vi "MP-285 GetSet Resolution.vi"(0 "VISA resource name":refnum<visa-resource-name>, 1 "Input: Resolution - H/L":string="\r", 2 "error in (no error)":errorcluster) -> (3 "VISA resource name 2":refnum<visa-resource-name>, 4 "Output: Resolution - H/L":string, 5 "Output: Resolution":bool, 6 "error out":errorcluster)   [LabVIEW 2010]
uses:
  StageMG100204SutterMP285/StageMG100204SutterMP285.lvclass
panel:
  out "Serial Read":string
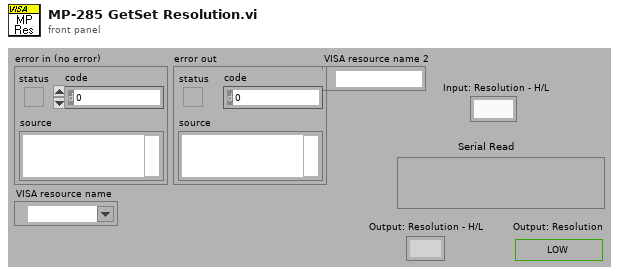
[diagram p1: front panel]
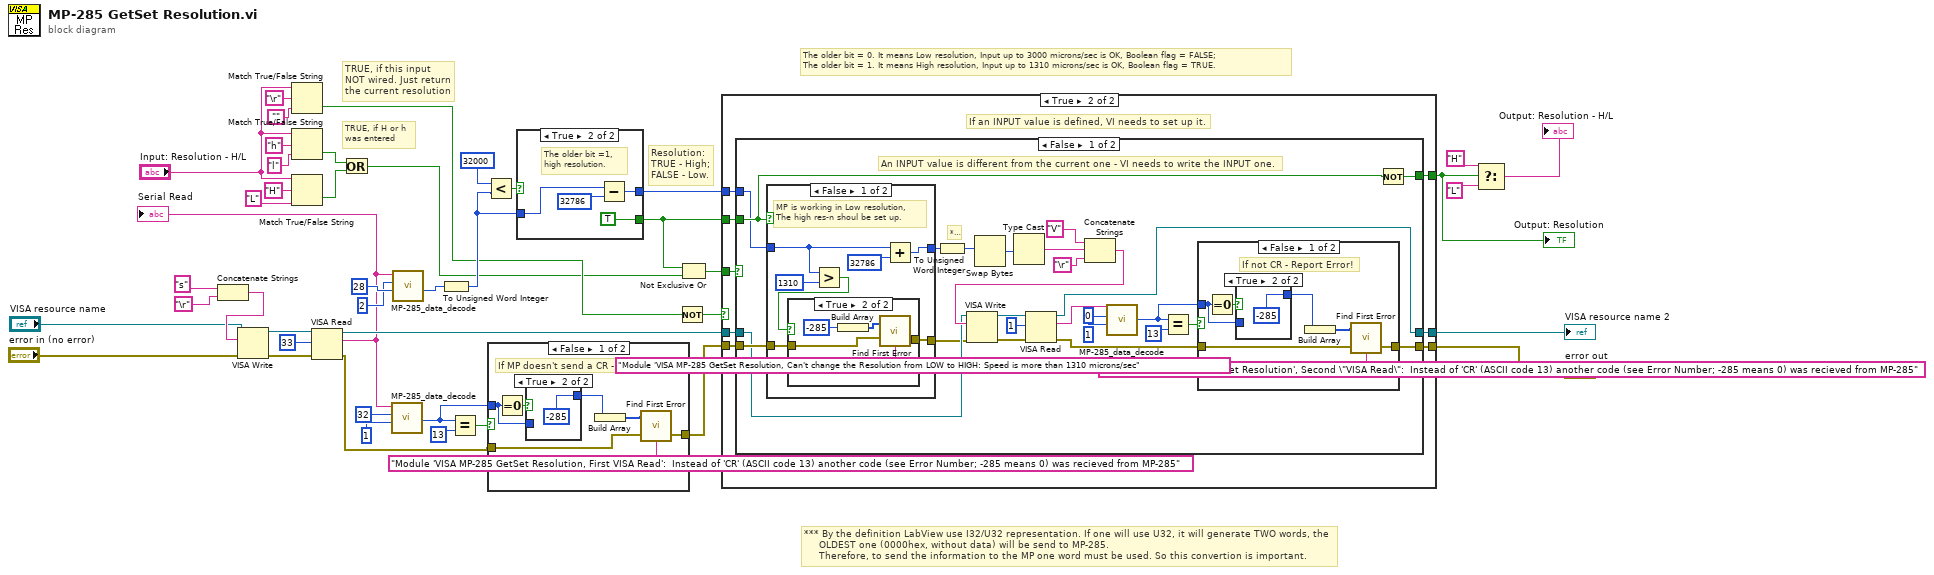
[diagram p0: block diagram]
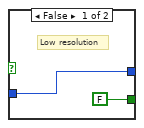
[diagram p8: hidden frame]
diagram:
  # "TRUE, if this input\nNOT wired. Just return\nthe current resolution"
  # "TRUE, if H or h\nwas entered"
  # "*** By the definition LabView use I32/U32 representation. If one will use U32, it will generate TWO words, the \n     OLDEST one (0000hex, without data) will be send to MP-285. \n     Therefore, to send the information to the MP one word must be used. So this convertion is important."
  # "The older bit = 0. It means Low resolution, Input up to 3000 microns/sec is OK, Boolean flag = FALSE;\nThe older bit = 1. It means High resolution, Input up to 1310 microns/sec is OK, Boolean flag = TRUE."
  # "Resolution:\nTRUE - High;\nFALSE - Low."
  n1 = Concatenate Strings("s", "\r") -> (w42:string)
  n2 = VISA Write(VISA resource name="VISA resource name", write buffer=w42, error in (no error)="error in (no error)") -> (VISA resource name out=w41:refnum<visa-resource-name>, error out=w40:errorcluster)  [unwired: 1 out]
  n3 = Match True/False String(2:"", 3:"\r", 4:"Input: Resolution - H/L") -> (0:w13:bool)  [unwired: 1 out]
  n4 = Match True/False String(2:"l", 3:"h", 4:"Input: Resolution - H/L") -> (0:w18:bool)  [unwired: 1 out]
  n5 = Match True/False String(2:"L", 3:"H", 4:"Input: Resolution - H/L") -> (0:w17:bool)  [unwired: 1 out]
  n6 = VISA Read(VISA resource name=w41, byte count=33, error in (no error)=w40) -> (VISA resource name out=w35:refnum<visa-resource-name>, read buffer=w22:string, error out=w30:errorcluster)  [unwired: 1 out]
  "Serial Read" <- w22
  n7 = Or(x=w18, y=w17) -> (x .or. y?=w11:bool)
  n8 = call "MP-285_data_decode.vi"("length"=32, "offset"=1, "encoded data string in"=w22) -> ("decoded data"=w36:i32)  [unwired: 6 in, 2 out]
  n9 = call "MP-285_data_decode.vi"("length"=28 ("offset (0)"), "offset"=2 ("length"), "encoded data string in"=w22) -> ("decoded data"=w32:i32)  [unwired: 6 in, 2 out]
  n10 = To Unsigned Word Integer(number=w32) -> (unsigned 16bit integer=w31:u16)
  n11 = Equal?(x=w36, y=13) -> (x = y?=w37:bool)
  n12 = Less?(x=32000, y=w31) -> (x < y?=w34:bool)
  n13 = case shown="False" w37 {
    tunnel: [w51 w54] -> w29
    tunnel: w36 -> [w47 _]
    tunnel: w30 -> [w45 w54]
    frame False {
      # "If MP doesn't send a CR - Report Error!"
      n14 = Equal To 0?(x=w47) -> (x = 0?=w48:bool)
      n15 = case shown="True" w48 {
        tunnel: w47 -> [w52 _]
        tunnel: [w52 -285] -> w46
        frame False {
        }
        frame True {
        }
      }
      n16 = Build Array(w46) -> (w49:i32[])
      n17 = call <vilib>:"Find First Error.vi"("error in (no error)"=w45, "source messages"="Module 'VISA MP-285 GetSet Resolution, First VISA Read':  Instead of 'CR' (ASCII code 13) another code (see Error Number; -285 means 0) was recieved from MP-285", "error codes"=w49) -> ("error out"=w51:errorcluster)  [unwired: 2 out]
    }
    frame True {
      # "TRUE: CR was received - NO Errors"
    }
  }
  n18 = case shown="True" w34 {
    tunnel: [w56 w60] -> w21
    tunnel: w31 -> [w56 w58]
    tunnel: [FALSE TRUE] -> w10
    frame False {
      # "Low resolution"
    }
    frame True {
      # "The older bit =1, \nhigh resolution."
      n19 = Subtract(x=w58, y=32786) -> (x-y=w60:i32)
    }
  }
  n20 = Not(x=w13) -> (.not. x?=w14:bool)
  n21 = Not Exclusive Or(1:w11, 2:w10) -> (0:w12:bool)
  n22 = case shown="True" w14 {
    tunnel: w35 -> [w63 w71]
    tunnel: w29 -> [w62 w70]
    tunnel: [w63 w69] -> w28
    tunnel: [w62 w68] -> w27
    tunnel: w10 -> [w61 w67]
    tunnel: w21 -> [_ w65]
    tunnel: w12 -> [_ w66]
    tunnel: [w61 w64] -> w3
    frame False {
      # "If an INPUT value was not seted up there is nothing to write, just output the current Resolution."
    }
    frame True {
      # "If an INPUT value is defined, VI needs to set up it."
      n23 = case shown="False" w66 {
        tunnel: w70 -> [w74 w124]
        tunnel: w71 -> [w73 w123]
        tunnel: [w87 w124] -> w68
        tunnel: [w81 w123] -> w69
        tunnel: w67 -> [w78 w122]
        tunnel: [w77 w122] -> w64
        tunnel: w65 -> [w76 _]
        frame False {
          # "***"
          # "An INPUT value is different from the current one - VI needs to write the INPUT one."
          n24 = case shown="False" w78 {
            tunnel: w76 -> [w111 w121]
            tunnel: [w113 w121] -> w84
            tunnel: w74 -> [w107 w120]
            tunnel: [w108 w120] -> w72
            frame False {
              # "MP is working in Low resolution,\nThe high res-n shoul be set up."
              n25 = Greater?(x=w111, y=1310) -> (0:w109:bool)
              n26 = case shown="True" w109 {
                tunnel: [w114 w116] -> w108
                tunnel: w107 -> [w114 w115]
                frame False {
                }
                frame True {
                  n27 = Build Array(-285) -> (w118:i32[])
                  n28 = call <vilib>:"Find First Error.vi"("error in (no error)"=w115, "source messages"="Module 'VISA MP-285 GetSet Resolution, Can't change the Resolution from LOW to HIGH: Speed is more than 1310 microns/sec", "error codes"=w118) -> ("error out"=w116:errorcluster)  [unwired: 2 out]
                }
              }
              n29 = Add(x=w111, y=32786) -> (x+y=w113:i32)
            }
            frame True {
              # "It is High resolution,\nLow resolution shoulb be\nset up."
            }
          }
          n30 = To Unsigned Word Integer(number=w84) -> (unsigned 16bit integer=w83:u16)
          n31 = Swap Bytes(anything=w83) -> (byte swapped=w86:u16)
          n32 = Type Cast(x=w86) -> (*(type *) &x=w85:string)  [unwired: 1 out]
          n33 = Concatenate Strings("V", w85, "\r") -> (w95:string)
          n34 = VISA Write(VISA resource name=w73, write buffer=w95, error in (no error)=w72) -> (VISA resource name out=w94:refnum<visa-resource-name>, error out=w93:errorcluster)  [unwired: 1 out]
          n35 = VISA Read(VISA resource name=w94, byte count=1, error in (no error)=w93) -> (VISA resource name out=w81:refnum<visa-resource-name>, read buffer=w82:string, error out=w75:errorcluster)  [unwired: 1 out]
          n36 = call "MP-285_data_decode.vi"("length"=0, "offset"=1, "encoded data string in"=w82) -> ("decoded data"=w88:i32)  [unwired: 6 in, 2 out]
          n37 = Equal?(x=w88, y=13) -> (x = y?=w89:bool)
          n38 = case shown="False" w89 {
            tunnel: [w103 w106] -> w87
            tunnel: w88 -> [w99 _]
            tunnel: w75 -> [w97 w106]
            frame False {
              # "If not CR - Report Error!"
              n39 = Equal To 0?(x=w99) -> (x = 0?=w100:bool)
              n40 = case shown="True" w100 {
                tunnel: w99 -> [w104 _]
                tunnel: [w104 -285] -> w98
                frame False {
                }
                frame True {
                }
              }
              n41 = Build Array(w98) -> (w101:i32[])
              n42 = call <vilib>:"Find First Error.vi"("error in (no error)"=w97, "source messages"="Module 'VISA MP-285 GetSet Resolution', Second \"VISA Read\":  Instead of 'CR' (ASCII code 13) another code (see Error Number; -285 means 0) was recieved from MP-285", "error codes"=w101) -> ("error out"=w103:errorcluster)  [unwired: 2 out]
            }
            frame True {
              # "TRUE CR was received - NO Errors"
            }
          }
          n43 = Not(x=w78) -> (.not. x?=w77:bool)
        }
        frame True {
          # "An INPUT value is the same, as current one --> Nothing to do!"
        }
      }
    }
  }
  "Output: Resolution" <- w3
  "VISA resource name 2" <- w28
  "error out" <- w27
  n44 = Select(t="H", s=w3, f="L") -> (s? t:f=→"Output: Resolution - H/L":string)
